vi "rolling resistance.vi"(9 "fr":dbl, 10 "g":dbl, 11 "Weight":dbl) -> (3 "result":dbl)   [LabVIEW 2014]
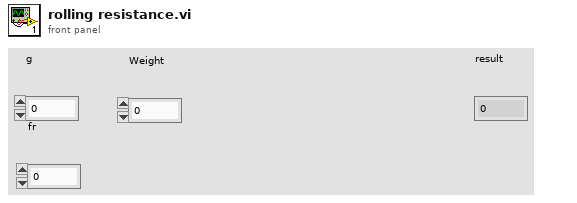
[diagram p1: front panel]
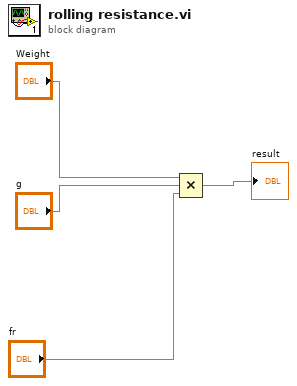
[diagram p0: block diagram]
diagram:
  n1 = Compound Arithmetic op=MULTIPLY("Weight", "g", "fr") -> (→"result":dbl)
